vi "top-level.vi"() -> ()   [LabVIEW 2014]
panel:
  out "XY Graph":cluster{i32[], dbl[]}(graph)
  out "Cluster":T1
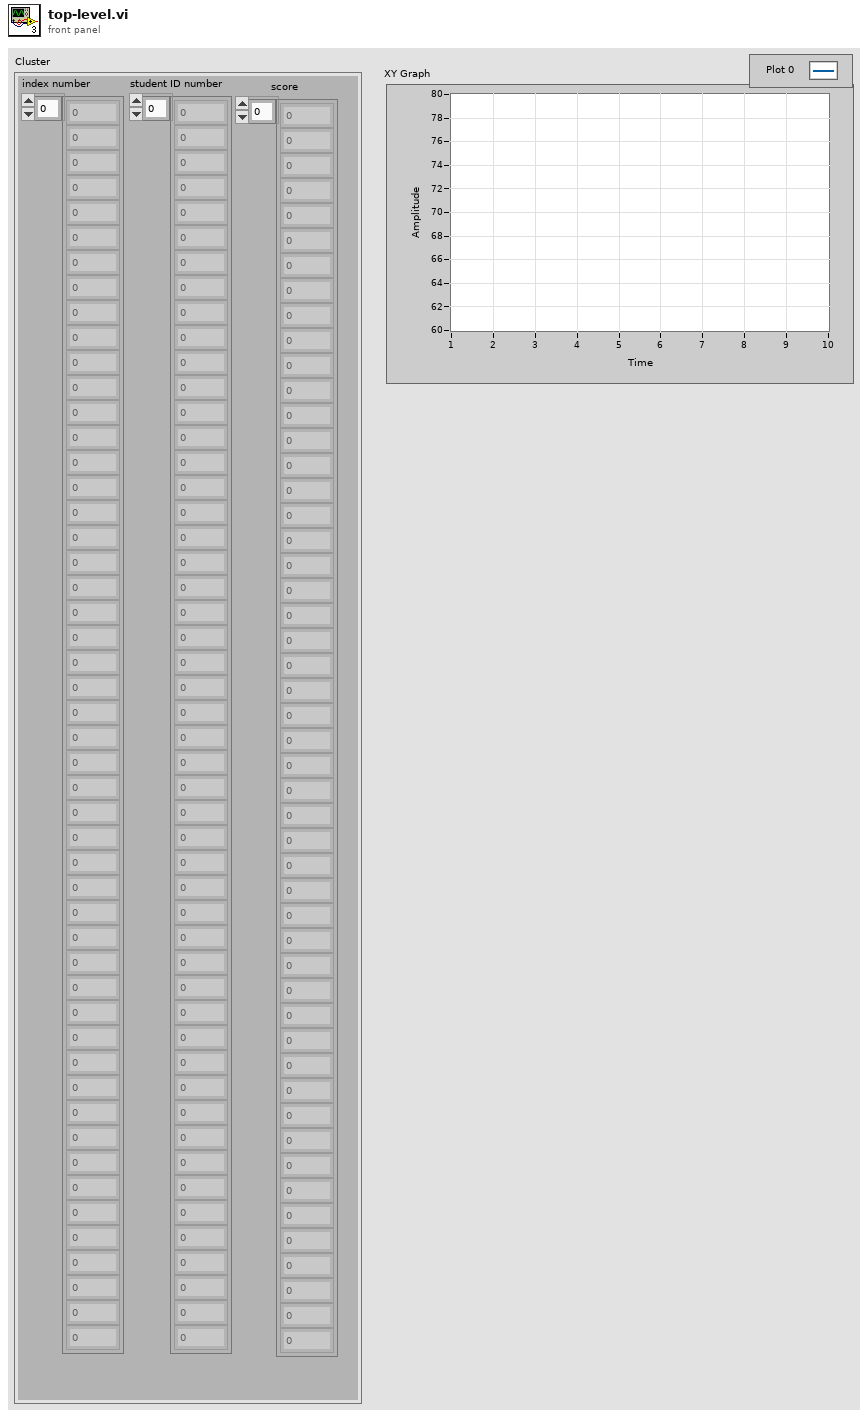
[diagram p1: front panel]
types:
  T1 = cluster{"index number":dbl[], "student ID number":dbl[], "score":dbl[]}
  T2 = cluster{"student ID number":dbl[], "score":dbl[]}
  T3 = cluster{i32[], "student ID number":dbl[], "score":dbl[]}
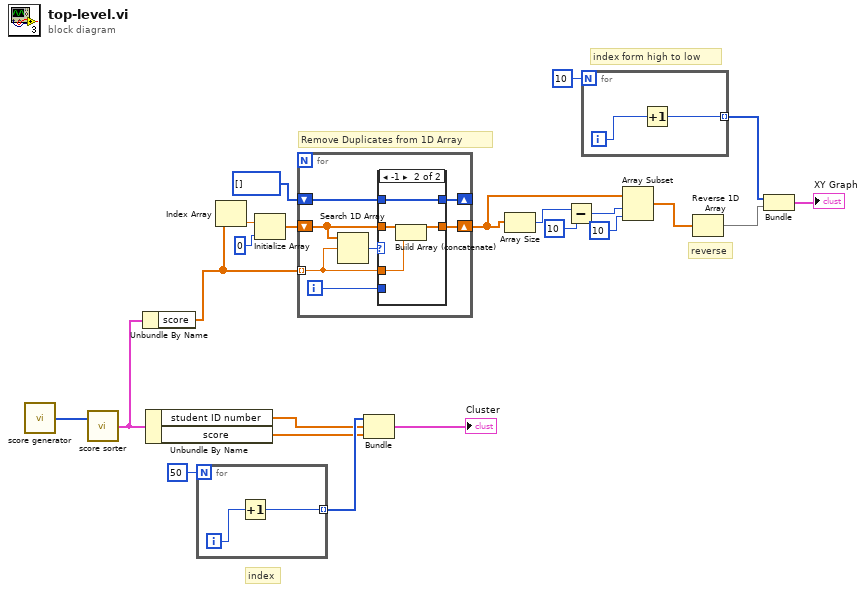
[diagram p0: block diagram]
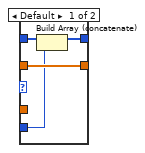
[diagram p2: hidden frame]
diagram:
  # "index"
  # "index form high to low"
  # "reverse"
  # "Remove Duplicates from 1D Array"
  n1 = call "score generator.vi"() -> ("Array"=w20:i32[])  [unwired: 4 in]
  n2 = call "score sorter.vi"("random score"=w20) -> ("Sorted Cluster"=w12:T2)  [unwired: 2 in]
  n3 = Unbundle By Name(w12) -> ("score"=w11:dbl[])
  n4 = Unbundle By Name(w12) -> ("student ID number"=w18:dbl[], "score"=w17:dbl[])
  n5 = for {
    N: 50 -> [_]
    tunnel: [w23] -> w21 mode=indexing
    i -> [w24]
    n6 = Increment(x=w24) -> (x+1=w23:i32)
  }
  n7 = Index Array(array=w11) -> (element=w15:dbl)  [unwired: 1 in]
  n8 = Initialize Array(w15, 0 ("Dimension Size")) -> (w14:dbl[])
  n9 = for {
    tunnel: w11 -> [w30] mode=indexing
    shift-right: [w29] -> w7
    shift-left: w14 -> [w28]
    shift-right: [w26] -> _
    shift-left: i32[] [] -> [w25]
    i -> [w27]
    n10 = Search 1D Array(1D array=w28, element=w30) -> (index of element=w31:i32)  [unwired: 1 in]
    n11 = case shown="-1" w31 {
      tunnel: w30 -> [_ w39]
      tunnel: [w35 w37] -> w29
      tunnel: w28 -> [w35 w38]
      tunnel: w27 -> [w32 _]
      tunnel: [w33 w36] -> w26
      tunnel: w25 -> [w34 w36]
      frame Default {
        n12 = Build Array (concatenate)(w34, w32) -> (w33:i32[])
      }
      frame -1 {
        n13 = Build Array (concatenate)(w38, w39) -> (w37:dbl[])
      }
    }
  }
  n14 = Bundle(w21, "student ID number"=w18, "score"=w17) -> (→"Cluster":T3)  [unwired: 1 in]
  n15 = Array Size(array=w7) -> (size(s)=w10:i32)
  n16 = Subtract(x=w10, y=10) -> (x-y=w8:i32)
  n17 = for {
    N: 10 -> [_]
    tunnel: [w40] -> w5 mode=indexing
    i -> [w41]
    n18 = Increment(x=w41) -> (x+1=w40:i32)
  }
  n19 = Array Subset(array=w7, index=w8, length=10) -> (w2:dbl[])
  n20 = Reverse 1D Array(array=w2) -> (reversed array=w1:dbl[])
  n21 = Bundle(w5, w1) -> (→"XY Graph":cluster{i32[], dbl[]})  [unwired: 1 in]
